vi "Bring_to_front.vi"(0 "path":path) -> ()   [LabVIEW 2010]
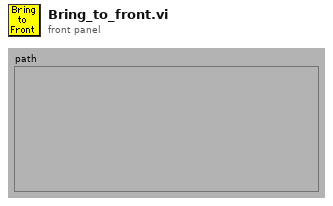
[diagram p1: front panel]
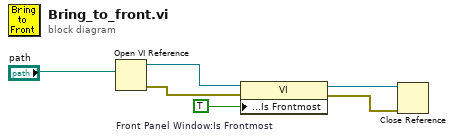
[diagram p0: block diagram]
diagram:
  w3 = TRUE  # Front Panel Window:Is Frontmost
  n1 = Open VI Reference(vi path="path") -> (vi reference=w5:refnum<vi>, error out=w4:errorcluster)  [unwired: 1 in, 4 out]
  n2 = property class="VI"(reference=w5, error in=w4, "Front Panel Window:Is Frontmost"=w3) -> (reference out=w2:refnum<vi>, error out=w1:errorcluster)
  n3 = Close Reference(reference=w2, error in (no error)=w1) -> ()  [unwired: 1 out]
